vi "New Namespace (Parent).vi"(8 "error in (no error)":errorcluster, 10 "New Namespace":string[](array[string]), 11 "BlueLogParent in":refnum<class "BlueLogParent_OpenSource.lvclass">) -> (0 "error out":errorcluster, 3 "BlueLogParent out":refnum<class "BlueLogParent_OpenSource.lvclass">)   [LabVIEW 2020, in "BlueLogParent_OpenSource.lvclass"]
uses:
  BlueLogParent_OpenSource.lvclass
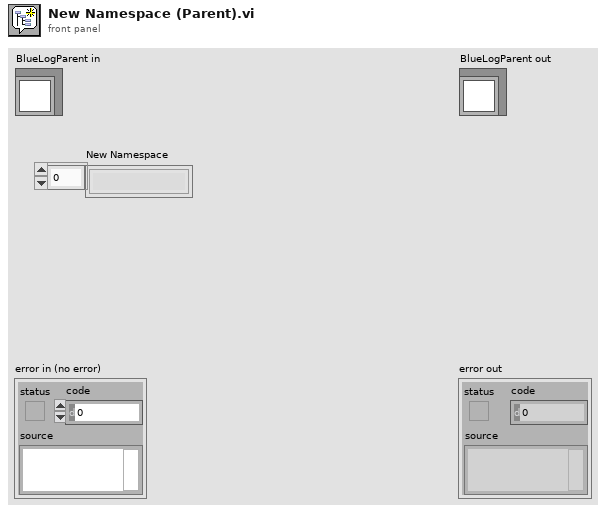
[diagram p1: front panel]
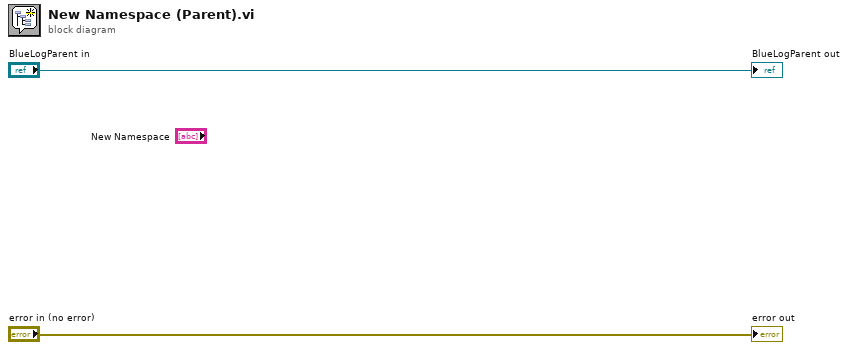
[diagram p0: block diagram]
diagram:
  "error out" <- "error in (no error)"
  "BlueLogParent out" <- "BlueLogParent in"
